vi "LHF.DB.Mongo.Collection.JSON.Find.vi"(6 "Extract _id":bool=TRUE, 8 "error in (no error)":errorcluster, 9 "query":variant, 10 "Collection":string, 11 "LHF.DB.Mongo in":refnum<class "LHF.DB.Mongo.lvclass">) -> (0 "error out":errorcluster, 1 "ObjectIDs":string[](array[string]), 2 "Documents":string[](array[string]), 3 "LHF.DB.Mongo out":refnum<class "LHF.DB.Mongo.lvclass">)   [LabVIEW 2013, in "LHF.DB.Mongo.lvclass"]
doc: "Query: use clusters named with query operation (if none, equal is used) or a Query.NET object. If a single field is being queried, you may it by setting the variable name as the field name in database. \nYou may use <, <=, >, >=, ==, !=, and others in variables name to choose operation, and you may aggregate them by putting in a cluster with $and or $or."
uses:
  LHF.DB.Mongo.lvclass
  C:/Users/Ricardo/Desktop/Projetos/LabVIEW-MongoDB/src/Driver/MongoDB.Driver.dll
  Driver/MongoDB.Driver.dll
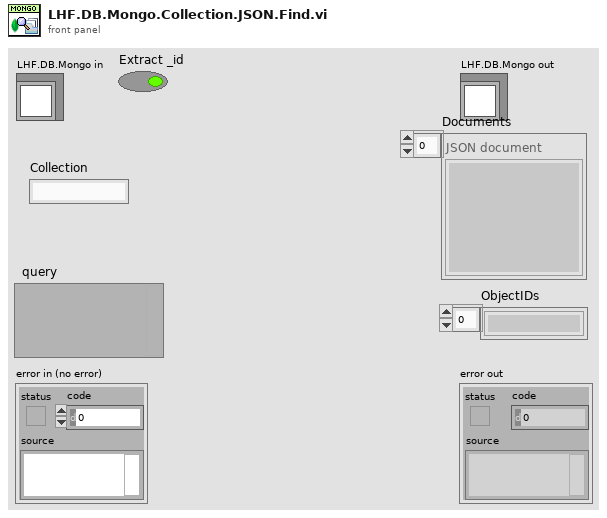
[diagram p1: front panel]
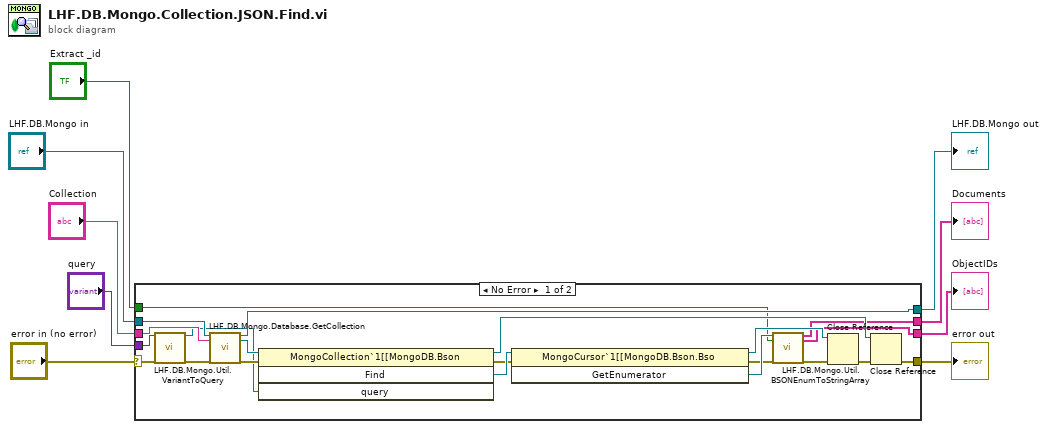
[diagram p0: block diagram]
diagram:
  n1 = case shown="No Error" "error in (no error)" {
    selector: "error in (no error)" -> [w17 w32]
    tunnel: [w22 w32] -> w8
    tunnel: [w29 w31] -> w6
    tunnel: "LHF.DB.Mongo in" -> [w28 w31]
    tunnel: "Collection" -> [w30 _]
    tunnel: [w14 _] -> w4
    tunnel: "query" -> [w20 _]
    tunnel: [w15 _] -> w2
    tunnel: "Extract _id" -> [w12 _]
    frame No Error {
      n2 = call "LHF.DB.Mongo.Util.VariantToQuery.vi"("Equal"=w20, "error in (no error)"=w17) -> (".NET Refnum out"=w18:refnum<k24>, "error out"=w16:errorcluster)  [unwired: 16 in]
      n3 = call "LHF.DB.Mongo.Database.GetCollection.vi"("LHF.DB.Mongo in"=w28, "collectionName"=w30, "error in (no error)"=w16) -> ("LHF.DB.Mongo in"=w29:refnum<class "LHF.DB.Mongo.lvclass">, "MongoCollection"=w21:refnum<k24>, "error out"=w19:errorcluster)  [unwired: 14 in]
      n4 = invoke class="MongoCollection`1[[MongoDB.Bson" method="Find"(reference=w21, error in=w19, "query"=w18) -> (reference out=w24:refnum<k24>, error out=w26:errorcluster, "Find"=w27:refnum<k24>)  [unwired: 1 in, 1 out]
      n5 = invoke class="MongoCursor`1[[MongoDB.Bson.Bso" method="GetEnumerator"(reference=w27, error in=w26) -> (reference out=w25:refnum<k24>, error out=w11:errorcluster, "GetEnumerator"=w13:refnum<k24>)  [unwired: 1 in]
      n6 = call "LHF.DB.Mongo.Util.BSONEnumToStringArray.vi"("BsonENUM"=w13, "Extract _id"=w12, "error in (no error)"=w11) -> ("Documents"=w14:string[], "_id Array"=w15:string[], "error out"=w10:errorcluster)  [unwired: 14 in]
      n7 = Close Reference(reference=w25, error in (no error)=w10) -> (error out=w23:errorcluster)
      n8 = Close Reference(reference=w24, error in (no error)=w23) -> (error out=w22:errorcluster)
    }
    frame Error {
    }
  }
  "error out" <- w8
  "LHF.DB.Mongo out" <- w6
  "Documents" <- w4
  "ObjectIDs" <- w2
